vi "Calculate_Servo_Angle(SubVI).vi"(10 "Multiplier":dbl=1.0, 11 "PrevServoAngle":dbl) -> (2 "Multiplier_out":dbl, 3 "ServoAngle":dbl)   [LabVIEW 2017]
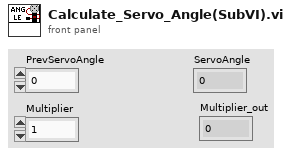
[diagram p1: front panel]
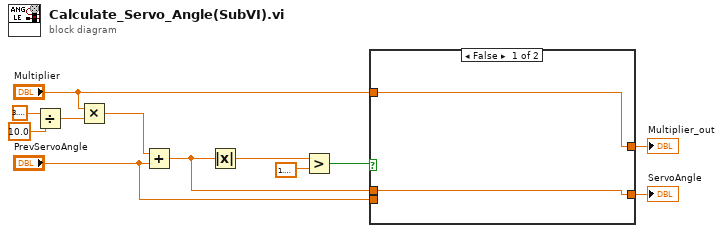
[diagram p0: block diagram]
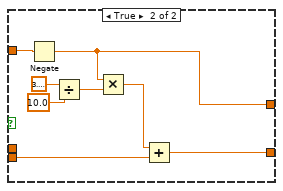
[diagram p2: hidden frame]
diagram:
  n1 = Divide(x=3.141592653589793, y=10.0) -> (x/y=w10:dbl)
  n2 = Multiply(x="Multiplier", y=w10) -> (x*y=w9:dbl)
  n3 = Add(x=w9, y="PrevServoAngle") -> (x+y=w1:dbl)
  n4 = Absolute Value(x=w1) -> (abs(x)=w7:dbl)
  n5 = Greater?(x=w7, y=1.5707963267948966) -> (0:w8:bool)
  n6 = case shown="False" w8 {
    tunnel: "Multiplier" -> [w14 w22]
    tunnel: [w14 w18] -> w4
    tunnel: "PrevServoAngle" -> [_ w17]
    tunnel: [w13 w15] -> w2
    tunnel: w1 -> [w13 _]
    frame False {
    }
    frame True {
      n7 = Negate(x=w22) -> (-x=w18:dbl)
      n8 = Divide(x=3.141592653589793, y=10.0) -> (x/y=w19:dbl)
      n9 = Multiply(x=w18, y=w19) -> (x*y=w16:dbl)
      n10 = Add(x=w16, y=w17) -> (x+y=w15:dbl)
    }
  }
  "Multiplier_out" <- w4
  "ServoAngle" <- w2
